vi "Enables.vi"() -> ()   [LabVIEW 2013]
panel:
  in  "Array":bool[](array[boolean])=[TRUE, TRUE, TRUE, TRUE, TRUE, TRUE, TRUE, TRUE, TRUE, TRUE, TRUE]
  in  "Rollers?":bool=TRUE
  in  "Intake?":bool=TRUE
  in  "Right Drive?":bool=TRUE
  in  "Left Drive?":bool=TRUE
  in  "Trigger?":bool=TRUE
  in  "Winch?":bool=TRUE
  in  "Arm?":bool=TRUE
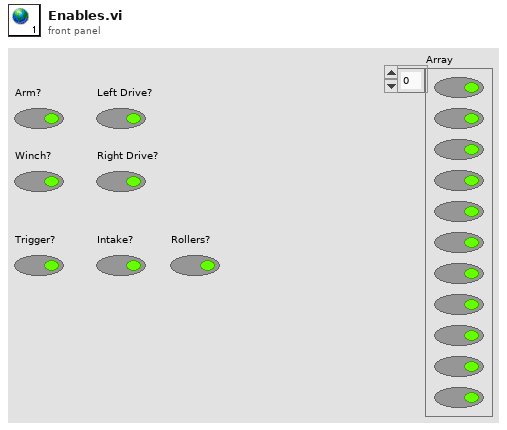
[diagram p1: front panel]
diagram:
